vi "findILCMap.vi"(8 "error in (no error)":errorcluster, 9 "Address":i32, 10 "Subnet":i32, 11 "ILCCommunications in":refnum<class "ILCCommunications.lvclass">) -> (0 "error out":errorcluster, 2 "Map":T1, 3 "ILCCommunications out":refnum<class "ILCCommunications.lvclass">)   [LabVIEW 2016, in "ILCCommunications.lvclass"]
uses:
  ILCCommunications.lvclass
  DataTypes/General/ILCMap.ctl
  DataTypes/General/ILCTypes.ctl
  ILCCommunications.lvclass/ILCCommunications.ctl
  DataTypes/General/M1M3SupportGeneral.lvlib
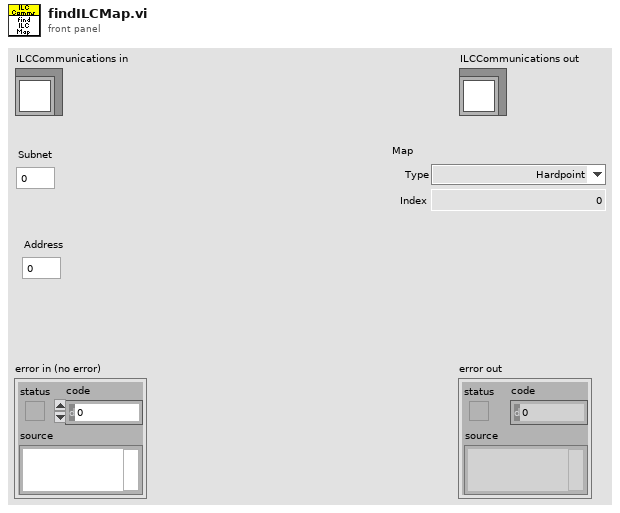
[diagram p1: front panel]
types:
  T1 = typedef "M1M3SupportGeneral.lvlib/ILCMap.ctl" = cluster{"Index":i32, "Type":T2}
  T2 = typedef "M1M3SupportGeneral.lvlib/ILCTypes.ctl" = enum16{"Hardpoint", "Force"}
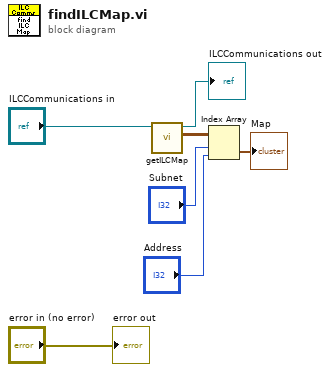
[diagram p0: block diagram]
diagram:
  n1 = call "getILCMap.vi"("ILCCommunications in"="ILCCommunications in") -> ("ILCMap"=w6:T1[][], "ILCCommunications out"=→"ILCCommunications out":refnum<class "ILCCommunications.lvclass">)  [unwired: 9 in]
  n2 = Index Array(array=w6, index (row)="Subnet", index (col)="Address") -> (element=→"Map":T1)
  "error out" <- "error in (no error)"
